vi "enableMotors.vi"(10 "Link 2 Demand":dbl, 11 "Link 1 Demand":dbl) -> (0 "Enable motor 2":bool, 1 "Enable motor 1":bool, 2 "Link 2 Demand 2":dbl, 3 "Link 1 Demand 2":dbl)   [LabVIEW 2017, in "admittanceControllerLibrary.lvlib"]
uses:
  admittanceControllerLibrary.lvlib
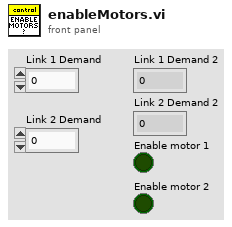
[diagram p1: front panel]
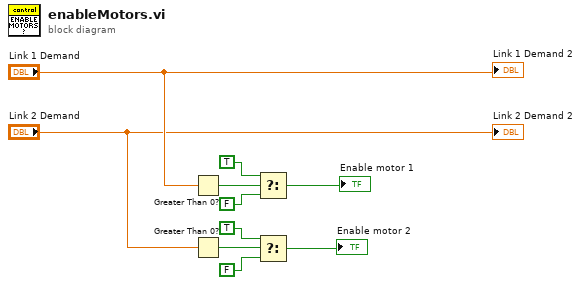
[diagram p0: block diagram]
diagram:
  n1 = Greater Than 0?(x="Link 1 Demand") -> (x > 0?=w8:bool)
  n2 = Greater Than 0?(x="Link 2 Demand") -> (x > 0?=w7:bool)
  n3 = Select(t=TRUE, s=w8, f=FALSE) -> (s? t:f=→"Enable motor 1":bool)
  n4 = Select(t=TRUE, s=w7, f=FALSE) -> (s? t:f=→"Enable motor 2":bool)
  "Link 1 Demand 2" <- "Link 1 Demand"
  "Link 2 Demand 2" <- "Link 2 Demand"
